vi "公式读取.vi"(8 "error in (no error)":errorcluster caption="错误输入（无错误）", 9 "量程":enum16{"低量程1", "低量程2", "高量程1", "高量程2"}(ring), 10 "测量模式":T1(ring), 11 "测量参数":enum16{"CODMn"}(ring)) -> (0 "error out":errorcluster caption="错误输出", 2 "临界滴定数":dbl format="%#_13g", 3 "公式":cluster{"X^2":dbl, "X":dbl, "b":dbl})   [LabVIEW 2016, in "斯坦道CODMn新电路板.lvlib"]
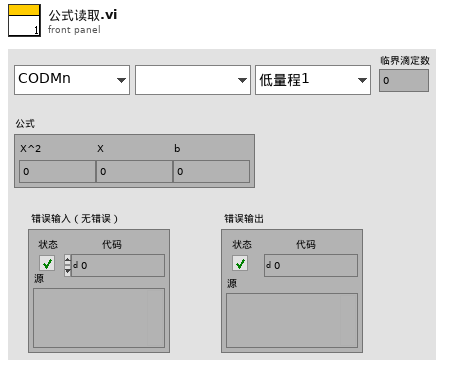
[diagram p1: front panel]
types:
  T1 = enum16{"", "水样测量", "标样核查", "零点核查", "跨度核查", "空白测试", "平行样测试", "加标回收"}
  T2 = cluster{"FLOAT[0]":sgl, "FLOAT[1]":sgl, "FLOAT[2]":sgl}
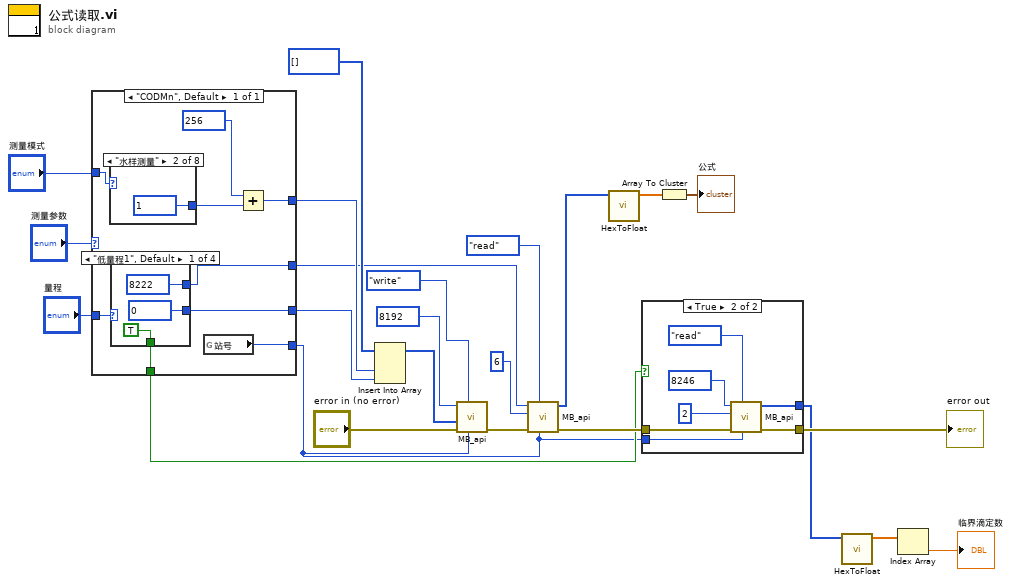
[diagram p0: block diagram]
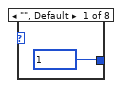
[diagram p3: hidden frame]
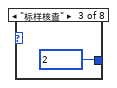
[diagram p4: hidden frame]
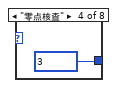
[diagram p5: hidden frame]
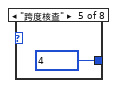
[diagram p6: hidden frame]
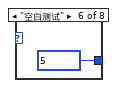
[diagram p7: hidden frame]
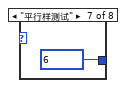
[diagram p8: hidden frame]
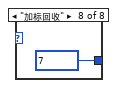
[diagram p9: hidden frame]
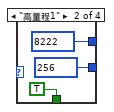
[diagram p10: hidden frame]
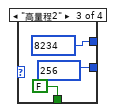
[diagram p11: hidden frame]
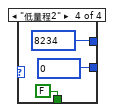
[diagram p12: hidden frame]
diagram:
  n1 = case shown="\"CODMn\", Default" "测量参数" {
    tunnel: "测量模式" -> [w27]
    tunnel: "量程" -> [w33]
    tunnel: [w29] -> w1
    tunnel: [w30] -> w17
    tunnel: [w32] -> w16
    tunnel: [w26] -> w8
    tunnel: [w25] -> w6
    frame "CODMn", Default {
      n2 = case shown="\"水样测量\"" w27 {
        tunnel: [u16 1 ("starting address") u16 1 ("starting address") u16 2 ("starting address") u16 3 ("starting address") u16 4 ("starting address") u16 5 ("starting address") u16 6 ("starting address") u16 7 ("starting address")] -> w28
        frame "", Default {
        }
        frame "水样测量" {
        }
        frame "标样核查" {
        }
        frame "零点核查" {
        }
        frame "跨度核查" {
        }
        frame "空白测试" {
        }
        frame "平行样测试" {
        }
        frame "加标回收" {
        }
      }
      n3 = case shown="\"低量程1\", Default" w33 {
        tunnel: [u16 0 ("starting address") u16 256 ("starting address") u16 256 ("starting address") u16 0 ("starting address")] -> w32
        tunnel: [u16 8222 ("starting address") u16 8222 ("starting address") u16 8234 ("starting address") u16 8234 ("starting address")] -> w26
        tunnel: [TRUE TRUE FALSE FALSE] -> w25
        frame "低量程1", Default {
        }
        frame "高量程1" {
        }
        frame "高量程2" {
        }
        frame "低量程2" {
        }
      }
      n4 = global read "CODMn断电保存全局变量.vi" "站号"() -> (w29:u16)
      n5 = Add(x=u16 256 ("starting address"), y=w28) -> (x+y=w30:u16)
    }
  }
  n6 = Insert Into Array(array=u16[] [] ("数组"), new element #1=w17, new element #2=w16) -> (w10:u16[])  [unwired: 1 in]
  n7 = call "MB_api.vi"("Slave ID"=w1, "STEP"=enum16{"open", "read", "write", "close"}."write", "Error in"="error in (no error)", "values"=w10, "starting address"=u16 8192) -> ("error out"=w13:errorcluster)  [unwired: 4 in, 2 out]
  n8 = call "MB_api.vi"("Slave ID"=w1, "STEP"=enum16{"open", "read", "write", "close"}."read", "Error in"=w13, "quantity"=u16 6, "starting address"=w8) -> ("error out"=w7:errorcluster, "Registers"=w21:u16[])  [unwired: 4 in, 1 out]
  n9 = call "HexToFloat.vi"("数组"=w21) -> ("FLOAT"=w20:sgl[])  [unwired: 10 in]
  n10 = case shown="True" w6 {
    tunnel: w7 -> [w54 w58]
    tunnel: [w54 w57] -> w5
    tunnel: [_ w56] -> w3
    tunnel: w1 -> [_ w55]
    frame False {
    }
    frame True {
      n11 = call "MB_api.vi"("Slave ID"=w55, "STEP"=enum16{"open", "read", "write", "close"}."read", "Error in"=w58, "quantity"=u16 2, "starting address"=u16 8246) -> ("error out"=w57:errorcluster, "Registers"=w56:u16[])  [unwired: 4 in, 1 out]
    }
  }
  "error out" <- w5
  n12 = Array To Cluster(array=w20) -> (cluster=→"公式":T2)
  n13 = call "HexToFloat.vi"("数组"=w3) -> ("FLOAT"=w2:sgl[])  [unwired: 10 in]
  n14 = Index Array(array=w2) -> (element=→"临界滴定数":sgl)  [unwired: 1 in]
